vi "UEGO sim component.vi"(5 "UEGO.1.negate":bool, 7 "UEGO.1.cal":bool, 10 "UEGO.1.lambda":fxp<+,12,3>=1.0, 11 "AI in":fxp<+/-,27,5> format="%.24g") -> (3 "AO out":fxp<+/-,37,21> format="%.23g")   [LabVIEW 2014]
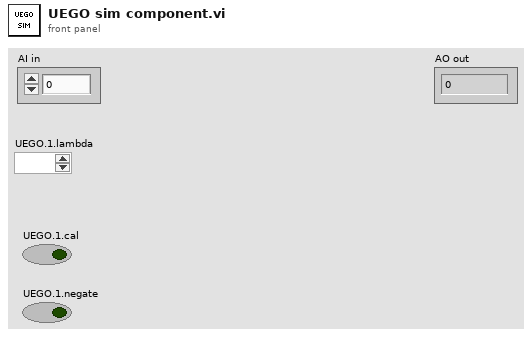
[diagram p1: front panel]
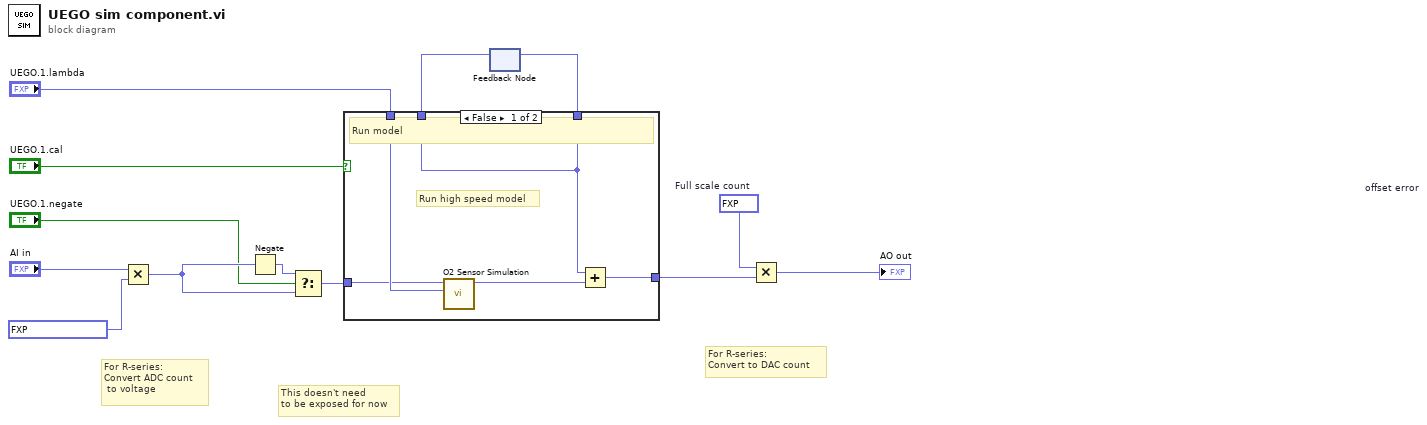
[diagram p0: block diagram]
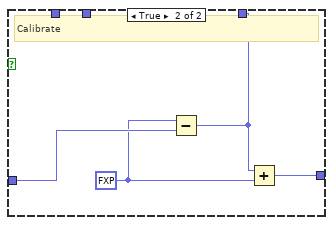
[diagram p2: hidden frame]
diagram:
  w4 = fxp<+,16,15> 3276.5  # Full scale count
  # "This doesn't need\nto be exposed for now"
  # "For R-series:\nConvert to DAC count"
  # "For R-series:\nConvert ADC count\n to voltage"
  n1 = Multiply(x="AI in", y=fxp<+,20,0> 0.00030517578125 ("input conversion")) -> (x*y=w8:fxp<+/-,47,5>)
  n2 = Negate(x=w8) -> (-x=w7:fxp<+/-,47,5>)
  n3 = Select(t=w7, s="UEGO.1.negate", f=w8) -> (s? t:f=w9:fxp<+/-,47,5>)
  n4 = feedback #1 "offset error"() -> (w1:fxp<+/-,49,7>)  [unwired: 1 in]
  n5 = case shown="False" "UEGO.1.cal" {
    tunnel: [w18 w20] -> w13
    tunnel: "UEGO.1.lambda" -> [w17 _]
    tunnel: w9 -> [w16 w22]
    tunnel: [w14 w19] -> w2
    tunnel: w1 -> [w14 _]
    frame False {
      # "Run high speed model"
      # "Run model"
      n6 = call "O2 Sensor Simulation.vi"("Lambda"=w17, "Voltage at Ip in"=w16) -> ("Vn Out"=w15:fxp<+/-,20,5>)  [unwired: 8 in, 1 out]
      n7 = Add(x=w14, y=w15) -> (x+y=w18:fxp<+/-,49,7>)
    }
    frame True {
      w21 = fxp<+/-,21,6> 0.5
      # "Calibrate"
      n8 = Subtract(x=w21, y=w22) -> (x-y=w19:fxp<+/-,49,7>)
      n9 = Add(x=w19, y=w21) -> (x+y=w20:fxp<+/-,50,8>)
    }
  }
  n10 = feedback-in #1(w2) -> ()
  n11 = Multiply(x=w4, y=w13) -> (x*y=→"AO out":fxp<+/-,64,23>)
